vi "GetLabVIEWInfos.vi"(8 "error in (no error)":errorcluster, 11 "application.lvclass":refnum<class "application.lvclass">) -> (0 "error out":errorcluster, 3 "application.lvclass (dup)":refnum<class "application.lvclass">)   [LabVIEW 2014, in "application.lvclass"]
uses:
  application.lvclass
  control/DEF-LabVIEW INFO.ctl
  application.lvclass/application.ctl
panel:
  out "LabVIEW Info":T1[](array[typedef])
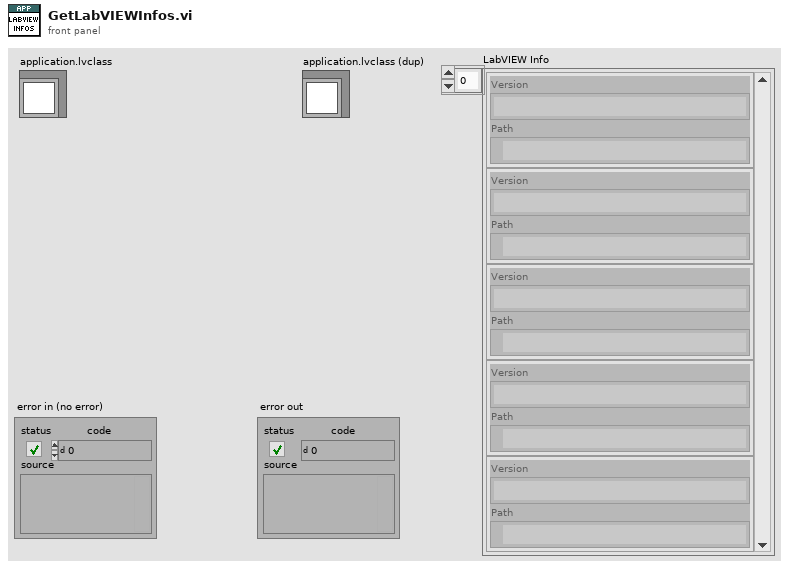
[diagram p1: front panel]
types:
  T1 = typedef "application.lvclass/DEF-LabVIEW INFO.ctl" = cluster{"Version":string, "Path":path}
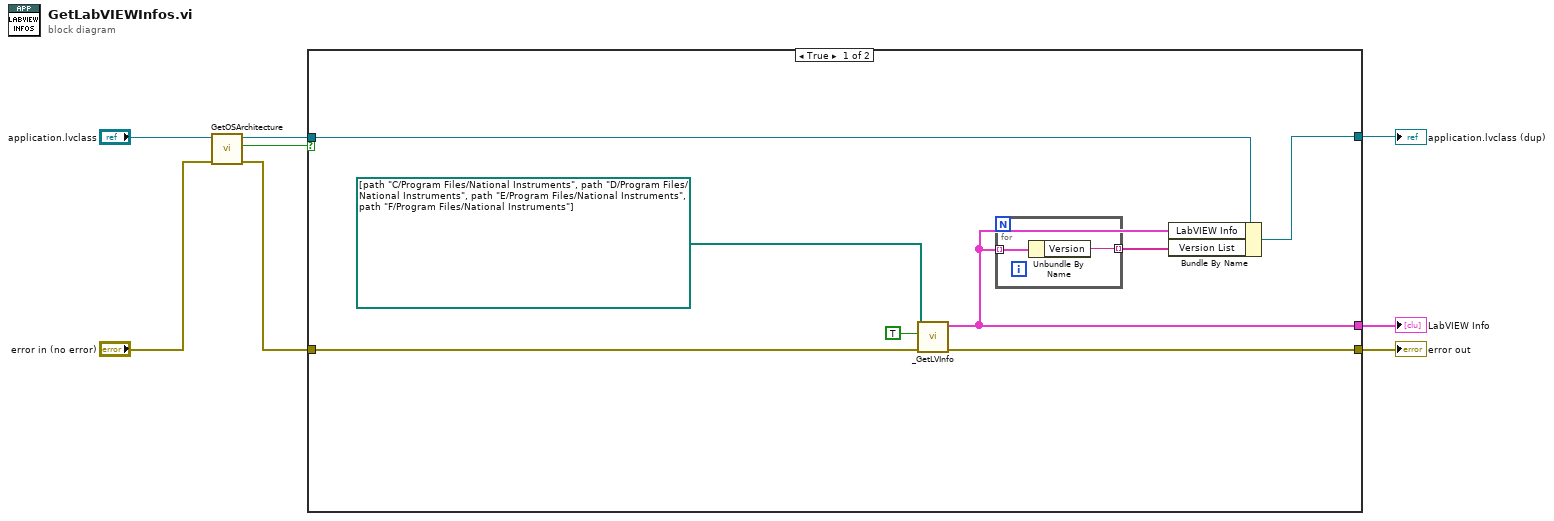
[diagram p0: block diagram]
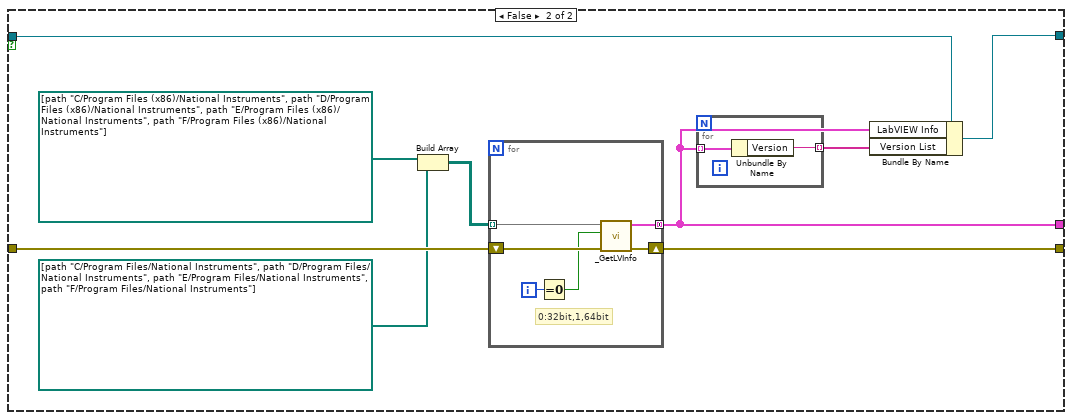
[diagram p2: hidden frame]
diagram:
  n1 = call "GetOSArchitecture.vi"("error in (no error)"="error in (no error)", "application in"="application.lvclass") -> ("error out"=w2:errorcluster, "32bit(T)/64bit(F)"=w1:bool, "application out"=w4:refnum<class "application.lvclass">)  [unwired: 7 in]
  n2 = case shown="True" w1 {
    tunnel: [w16 w27] -> w8
    tunnel: [w14 w25] -> w7
    tunnel: [w13 w24] -> w5
    tunnel: w4 -> [w12 w23]
    tunnel: w2 -> [w11 w22]
    frame True {
      n3 = call "_GetLVInfo.vi"("error in (no error)"=w11, "32bit(T)/64bit(F)"=TRUE, "Array"=path[] [path "C:/Program Files/National Instruments", path "D:/Program Files/National Instruments", path "E:/Program Files/National Instruments", path "F:/Program Files/National Instruments"]) -> ("error out"=w16:errorcluster, "LabVIEW Info"=w14:T1[])  [unwired: 7 in]
      n4 = for {
        tunnel: w14 -> [w18] mode=indexing
        tunnel: [w17] -> w15 mode=indexing
        n5 = Unbundle By Name(w18) -> ("Version"=w17:string)
      }
      n6 = Bundle By Name(cluster=w12, "LabVIEW Info"=w14, "Version List"=w15) -> (w13:refnum<class "application.lvclass">)
    }
    frame False {
      n7 = Build Array(path[] [path "C:/Program Files (x86)/National Instruments", path "D:/Program Files (x86)/National Instruments", path "E:/Program Files (x86)/National Instruments", path "F:/Program Files (x86)/National Instruments"], path[] [path "C:/Program Files/National Instruments", path "D:/Program Files/National Instruments", path "E:/Program Files/National Instruments", path "F:/Program Files/National Instruments"]) -> (w19:path[][])
      n8 = for {
        tunnel: [w32] -> w25 mode=concatenating
        shift-right: [w33] -> w27
        shift-left: w22 -> [w31]
        tunnel: w19 -> [w30] mode=indexing
        i -> [w29]
        # "0:32bit,1,64bit"
        n9 = Equal To 0?(x=w29) -> (x = 0?=w28:bool)
        n10 = call "_GetLVInfo.vi"("error in (no error)"=w31, "32bit(T)/64bit(F)"=w28, "Array"=w30) -> ("error out"=w33:errorcluster, "LabVIEW Info"=w32:T1[])  [unwired: 7 in]
      }
      n11 = for {
        tunnel: w25 -> [w35] mode=indexing
        tunnel: [w34] -> w26 mode=indexing
        n12 = Unbundle By Name(w35) -> ("Version"=w34:string)
      }
      n13 = Bundle By Name(cluster=w23, "LabVIEW Info"=w25, "Version List"=w26) -> (w24:refnum<class "application.lvclass">)
    }
  }
  "LabVIEW Info" <- w7
  "error out" <- w8
  "application.lvclass (dup)" <- w5
